vi "Read an digital IO desc.vi"(7 "Variable Defenition":T1) -> (4 "Header":string, 8 "concatenated string":string)   [LabVIEW 2011]
uses:
  Measurments Handling/Fixed Digital Channel Definition.ctl
  Measurments Handling/Update frequensies.ctl
  Measurments Handling/Channel catagory Enum.ctl
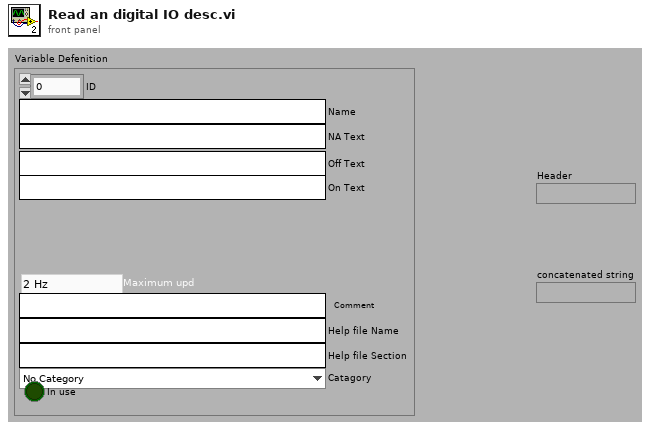
[diagram p1: front panel]
types:
  T1 = typedef "Fixed Digital Channel Definition.ctl" = cluster{"ID":u16, "Name":string, "NA Text":string, "Off Text":string, "On Text":string, "Maximum upd":T2, "Comment":string, "Help file Name":string, "Help file Section ":string, "Catagory":T3, "In use":bool}
  T2 = typedef "Update frequensies.ctl" = enum16{"2 Hz", "1 Hz", "0.1 Hz"}
  T3 = typedef "Channel catagory Enum.ctl" = enum16{"No Category", "Power", "Temperature", "Pressure"}
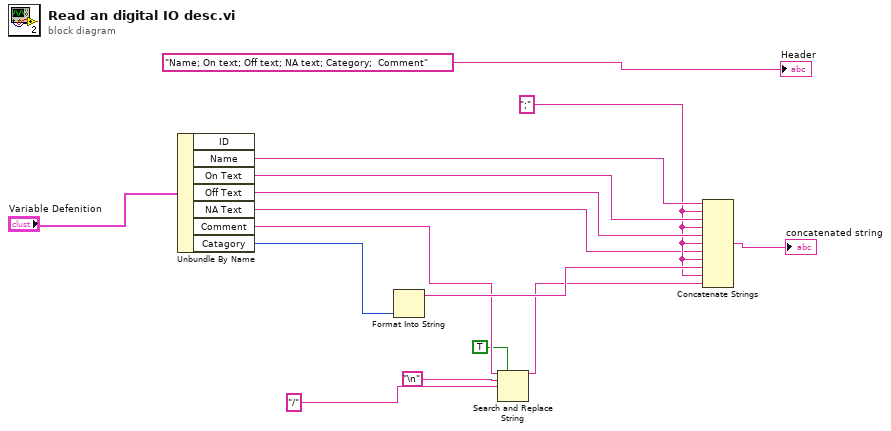
[diagram p0: block diagram]
diagram:
  w7 = ";" ("string")
  n1 = Unbundle By Name("Variable Defenition") -> ("Name"=w10:string, "On Text"=w9:string, "Off Text"=w8:string, "NA Text"=w6:string, "Comment"=w5:string, "Catagory"=w15:T3)  [unwired: 1 out]
  n2 = Format Into String(w15) -> (resulting string=w14:string)  [unwired: 3 in, 1 out]
  n3 = Search and Replace String(replace all?=TRUE ("replace all? (F)"), input string=w5, search string="\n", replace string="/" ("replace string (\"\")")) -> (result string=w4:string)  [unwired: 4 in, 3 out]
  n4 = Concatenate Strings(w10, w7, w9, w7, w8, w7, w6, w7, w14, w7, w4) -> (→"concatenated string":string)
  "Header" <- "Name; On text; Off text; NA text; Category;  Comment" ("Header")
